vi "Binary Clock 2012 NIVerified - Cópia.vi"() -> ()   [LabVIEW 2018]
doc: "This VI displays an ultimate digital watch, which is also known as binary clock."
panel:
  out "Boolean 4":bool
  out "Boolean 3":bool
  out "Boolean 2":bool
  out "Boolean":bool
  out "'a'33 3":bool
  out "'b'33 3":bool
  out "'c'33 3":bool
  out "'d'33 3":bool
  out "'e'33 3":bool
  out "'g'33 3":bool
  out "'f'33 3":bool
  out "'a'33 2":bool
  out "'b'33 2":bool
  out "'c'33 2":bool
  out "'d'33 2":bool
  out "'e'33 2":bool
  out "'g'33 2":bool
  out "'f'33 2":bool
  out "'a'33":bool
  out "'b'33":bool
  out "'c'33":bool
  out "'d'33":bool
  out "'e'33":bool
  out "'g'33":bool
  out "'f'33":bool
  out "'a'33":bool
  out "'b'33":bool
  out "'c'33":bool
  out "'d'33":bool
  out "'e'33":bool
  out "'g'33":bool
  out "'f'33":bool
  out "'a'3 2":bool
  out "'b'3 2":bool
  out "'c'3 2":bool
  out "'d'3 2":bool
  out "'e'3 2":bool
  out "'g'3 2":bool
  out "'f'3 2":bool
  out "'e'3":bool
  out "'f'3":bool
  out "'c'3":bool
  out "'b'3":bool
  out "'d'3":bool
  out "'g'3":bool
  out "'a'3":bool
  in  "stop":bool
  in  "Lap":bool
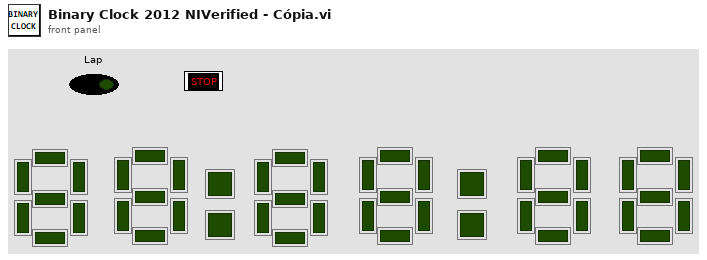
[diagram p1: front panel]
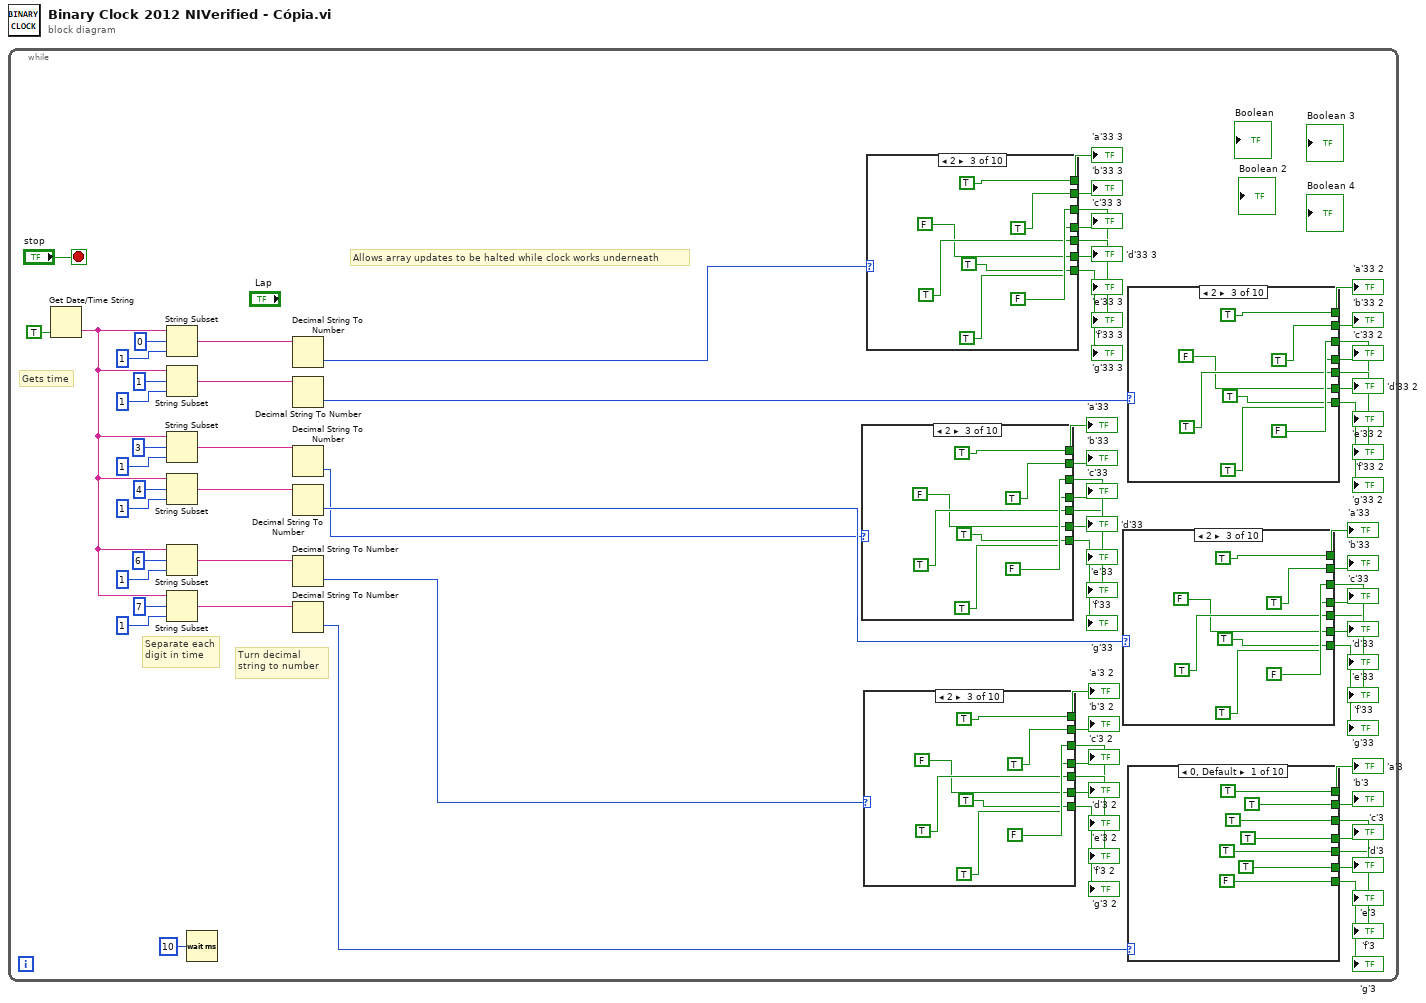
[diagram p0: block diagram]
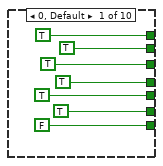
[diagram p2: hidden frame]
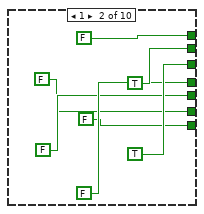
[diagram p3: hidden frame]
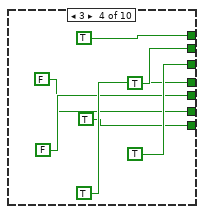
[diagram p4: hidden frame]
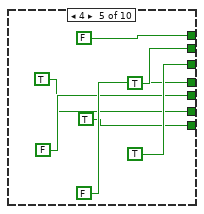
[diagram p5: hidden frame]
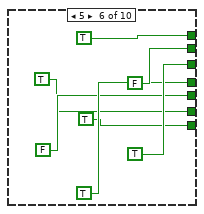
[diagram p6: hidden frame]
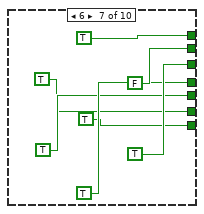
[diagram p7: hidden frame]
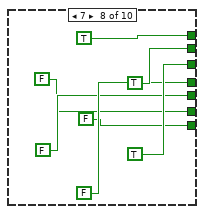
[diagram p8: hidden frame]
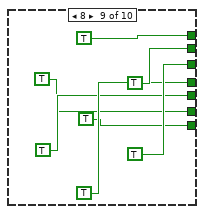
[diagram p9: hidden frame]
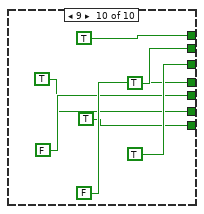
[diagram p10: hidden frame]
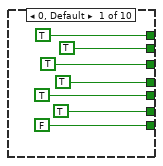
[diagram p11: hidden frame]
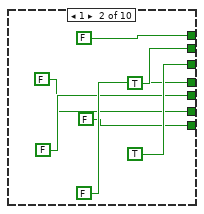
[diagram p12: hidden frame]
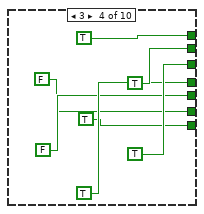
[diagram p13: hidden frame]
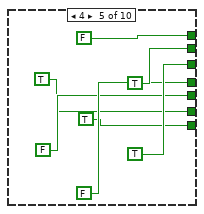
[diagram p14: hidden frame]
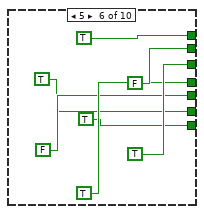
[diagram p15: hidden frame]
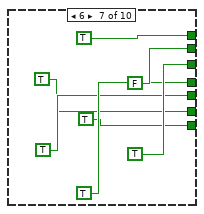
[diagram p16: hidden frame]
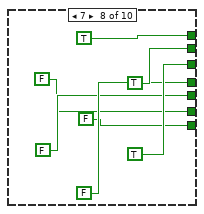
[diagram p17: hidden frame]
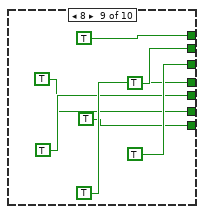
[diagram p18: hidden frame]
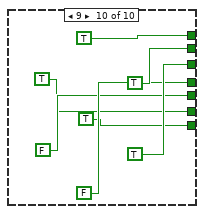
[diagram p19: hidden frame]
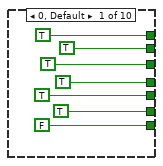
[diagram p20: hidden frame]
diagram:
  n1 = while {
    stop <- "stop" stop-if-true
    # "Allows array updates to be halted while clock works underneath"
    # "Turn decimal \nstring to number"
    # "Separate each\ndigit in time"
    # "Gets time"
    n2 = Get Date/Time String(want seconds? (F)=TRUE) -> (time string=w57:string)  [unwired: 2 in, 1 out]
    n3 = String Subset(string=w57, offset (0)=0, length (rest)=1 ("length (rest)")) -> (substring=w56:string)
    n4 = String Subset(string=w57, offset (0)=1, length (rest)=1 ("length (rest)")) -> (substring=w55:string)
    n5 = String Subset(string=w57, offset (0)=3, length (rest)=1 ("length (rest)")) -> (substring=w54:string)
    n6 = String Subset(string=w57, offset (0)=4, length (rest)=1 ("length (rest)")) -> (substring=w53:string)
    n7 = String Subset(string=w57, offset (0)=6, length (rest)=1 ("length (rest)")) -> (substring=w52:string)
    n8 = String Subset(string=w57, offset (0)=7, length (rest)=1 ("length (rest)")) -> (substring=w51:string)
    n9 = Wait (ms)(milliseconds to wait=u32 10) -> ()  [unwired: 1 out]
    n10 = Decimal String To Number(string=w56) -> (number=w1:i32)  [unwired: 2 in, 1 out]
    n11 = Decimal String To Number(string=w55) -> (number=w2:i32)  [unwired: 2 in, 1 out]
    n12 = Decimal String To Number(string=w54) -> (number=w3:i32)  [unwired: 2 in, 1 out]
    n13 = Decimal String To Number(string=w53) -> (number=w4:i32)  [unwired: 2 in, 1 out]
    n14 = Decimal String To Number(string=w52) -> (number=w33:i32)  [unwired: 2 in, 1 out]
    n15 = Decimal String To Number(string=w51) -> (number=w41:i32)  [unwired: 2 in, 1 out]
    n16 = case shown="2" w3 {
      tunnel: [TRUE ("'a'3") FALSE ("'a'3") TRUE ("'a'3") TRUE ("'a'3") FALSE ("'a'3") TRUE ("'a'3") TRUE ("'a'3") TRUE ("'a'3") TRUE ("'a'3") TRUE ("'a'3")] -> w25
      tunnel: [TRUE ("'a'3") TRUE ("'a'3") TRUE ("'a'3") TRUE ("'a'3") TRUE ("'a'3") FALSE ("'a'3") FALSE ("'a'3") TRUE ("'a'3") TRUE ("'a'3") TRUE ("'a'3")] -> w24
      tunnel: [TRUE ("'a'3") TRUE ("'a'3") FALSE ("'a'3") TRUE ("'a'3") TRUE ("'a'3") TRUE ("'a'3") TRUE ("'a'3") TRUE ("'a'3") TRUE ("'a'3") TRUE ("'a'3")] -> w23
      tunnel: [TRUE ("'a'3") FALSE ("'a'3") TRUE ("'a'3") TRUE ("'a'3") FALSE ("'a'3") TRUE ("'a'3") TRUE ("'a'3") FALSE ("'a'3") TRUE ("'a'3") FALSE ("'a'3")] -> w22
      tunnel: [TRUE ("'a'3") FALSE ("'a'3") TRUE ("'a'3") FALSE ("'a'3") FALSE ("'a'3") FALSE ("'a'3") TRUE ("'a'3") FALSE ("'a'3") TRUE ("'a'3") FALSE ("'a'3")] -> w21
      tunnel: [FALSE ("'a'3") FALSE ("'a'3") TRUE ("'a'3") TRUE ("'a'3") TRUE ("'a'3") TRUE ("'a'3") TRUE ("'a'3") FALSE ("'a'3") TRUE ("'a'3") TRUE ("'a'3")] -> w20
      tunnel: [TRUE ("'a'3") FALSE ("'a'3") FALSE ("'a'3") FALSE ("'a'3") TRUE ("'a'3") TRUE ("'a'3") TRUE ("'a'3") FALSE ("'a'3") TRUE ("'a'3") TRUE ("'a'3")] -> w19
      frame 0, Default {
      }
      frame 1 {
      }
      frame 2 {
      }
      frame 3 {
      }
      frame 4 {
      }
      frame 5 {
      }
      frame 6 {
      }
      frame 7 {
      }
      frame 8 {
      }
      frame 9 {
      }
    }
    "'a'33" <- w25
    "'b'33" <- w24
    "'c'33" <- w23
    "'d'33" <- w22
    "'e'33" <- w21
    "'g'33" <- w20
    "'f'33" <- w19
    n17 = case shown="2" w33 {
      tunnel: [TRUE ("'a'3") FALSE ("'a'3") TRUE ("'a'3") TRUE ("'a'3") FALSE ("'a'3") TRUE ("'a'3") TRUE ("'a'3") TRUE ("'a'3") TRUE ("'a'3") TRUE ("'a'3")] -> w34
      tunnel: [TRUE ("'a'3") TRUE ("'a'3") TRUE ("'a'3") TRUE ("'a'3") TRUE ("'a'3") FALSE ("'a'3") FALSE ("'a'3") TRUE ("'a'3") TRUE ("'a'3") TRUE ("'a'3")] -> w35
      tunnel: [TRUE ("'a'3") TRUE ("'a'3") FALSE ("'a'3") TRUE ("'a'3") TRUE ("'a'3") TRUE ("'a'3") TRUE ("'a'3") TRUE ("'a'3") TRUE ("'a'3") TRUE ("'a'3")] -> w36
      tunnel: [TRUE ("'a'3") FALSE ("'a'3") TRUE ("'a'3") TRUE ("'a'3") FALSE ("'a'3") TRUE ("'a'3") TRUE ("'a'3") FALSE ("'a'3") TRUE ("'a'3") FALSE ("'a'3")] -> w37
      tunnel: [TRUE ("'a'3") FALSE ("'a'3") TRUE ("'a'3") FALSE ("'a'3") FALSE ("'a'3") FALSE ("'a'3") TRUE ("'a'3") FALSE ("'a'3") TRUE ("'a'3") FALSE ("'a'3")] -> w38
      tunnel: [FALSE ("'a'3") FALSE ("'a'3") TRUE ("'a'3") TRUE ("'a'3") TRUE ("'a'3") TRUE ("'a'3") TRUE ("'a'3") FALSE ("'a'3") TRUE ("'a'3") TRUE ("'a'3")] -> w39
      tunnel: [TRUE ("'a'3") FALSE ("'a'3") FALSE ("'a'3") FALSE ("'a'3") TRUE ("'a'3") TRUE ("'a'3") TRUE ("'a'3") FALSE ("'a'3") TRUE ("'a'3") TRUE ("'a'3")] -> w40
      frame 0, Default {
      }
      frame 1 {
      }
      frame 2 {
      }
      frame 3 {
      }
      frame 4 {
      }
      frame 5 {
      }
      frame 6 {
      }
      frame 7 {
      }
      frame 8 {
      }
      frame 9 {
      }
    }
    "'a'3 2" <- w34
    "'b'3 2" <- w35
    "'c'3 2" <- w36
    "'d'3 2" <- w37
    "'e'3 2" <- w38
    "'g'3 2" <- w39
    "'f'3 2" <- w40
    n18 = case shown="2" w1 {
      tunnel: [TRUE ("'a'3") FALSE ("'a'3") TRUE ("'a'3") TRUE ("'a'3") FALSE ("'a'3") TRUE ("'a'3") TRUE ("'a'3") TRUE ("'a'3") TRUE ("'a'3") TRUE ("'a'3")] -> w5
      tunnel: [TRUE ("'a'3") TRUE ("'a'3") TRUE ("'a'3") TRUE ("'a'3") TRUE ("'a'3") FALSE ("'a'3") FALSE ("'a'3") TRUE ("'a'3") TRUE ("'a'3") TRUE ("'a'3")] -> w6
      tunnel: [TRUE ("'a'3") TRUE ("'a'3") FALSE ("'a'3") TRUE ("'a'3") TRUE ("'a'3") TRUE ("'a'3") TRUE ("'a'3") TRUE ("'a'3") TRUE ("'a'3") TRUE ("'a'3")] -> w7
      tunnel: [TRUE ("'a'3") FALSE ("'a'3") TRUE ("'a'3") TRUE ("'a'3") FALSE ("'a'3") TRUE ("'a'3") TRUE ("'a'3") FALSE ("'a'3") TRUE ("'a'3") FALSE ("'a'3")] -> w8
      tunnel: [TRUE ("'a'3") FALSE ("'a'3") TRUE ("'a'3") FALSE ("'a'3") FALSE ("'a'3") FALSE ("'a'3") TRUE ("'a'3") FALSE ("'a'3") TRUE ("'a'3") FALSE ("'a'3")] -> w9
      tunnel: [FALSE ("'a'3") FALSE ("'a'3") TRUE ("'a'3") TRUE ("'a'3") TRUE ("'a'3") TRUE ("'a'3") TRUE ("'a'3") FALSE ("'a'3") TRUE ("'a'3") TRUE ("'a'3")] -> w10
      tunnel: [TRUE ("'a'3") FALSE ("'a'3") FALSE ("'a'3") FALSE ("'a'3") TRUE ("'a'3") TRUE ("'a'3") TRUE ("'a'3") FALSE ("'a'3") TRUE ("'a'3") TRUE ("'a'3")] -> w11
      frame 0, Default {
      }
      frame 1 {
      }
      frame 2 {
      }
      frame 3 {
      }
      frame 4 {
      }
      frame 5 {
      }
      frame 6 {
      }
      frame 7 {
      }
      frame 8 {
      }
      frame 9 {
      }
    }
    "'a'33 3" <- w5
    "'b'33 3" <- w6
    "'c'33 3" <- w7
    "'d'33 3" <- w8
    "'e'33 3" <- w9
    "'g'33 3" <- w10
    "'f'33 3" <- w11
    n19 = case shown="2" w4 {
      tunnel: [TRUE ("'a'3") FALSE ("'a'3") TRUE ("'a'3") TRUE ("'a'3") FALSE ("'a'3") TRUE ("'a'3") TRUE ("'a'3") TRUE ("'a'3") TRUE ("'a'3") TRUE ("'a'3")] -> w32
      tunnel: [TRUE ("'a'3") TRUE ("'a'3") TRUE ("'a'3") TRUE ("'a'3") TRUE ("'a'3") FALSE ("'a'3") FALSE ("'a'3") TRUE ("'a'3") TRUE ("'a'3") TRUE ("'a'3")] -> w31
      tunnel: [TRUE ("'a'3") TRUE ("'a'3") FALSE ("'a'3") TRUE ("'a'3") TRUE ("'a'3") TRUE ("'a'3") TRUE ("'a'3") TRUE ("'a'3") TRUE ("'a'3") TRUE ("'a'3")] -> w30
      tunnel: [TRUE ("'a'3") FALSE ("'a'3") TRUE ("'a'3") TRUE ("'a'3") FALSE ("'a'3") TRUE ("'a'3") TRUE ("'a'3") FALSE ("'a'3") TRUE ("'a'3") FALSE ("'a'3")] -> w29
      tunnel: [TRUE ("'a'3") FALSE ("'a'3") TRUE ("'a'3") FALSE ("'a'3") FALSE ("'a'3") FALSE ("'a'3") TRUE ("'a'3") FALSE ("'a'3") TRUE ("'a'3") FALSE ("'a'3")] -> w28
      tunnel: [FALSE ("'a'3") FALSE ("'a'3") TRUE ("'a'3") TRUE ("'a'3") TRUE ("'a'3") TRUE ("'a'3") TRUE ("'a'3") FALSE ("'a'3") TRUE ("'a'3") TRUE ("'a'3")] -> w27
      tunnel: [TRUE ("'a'3") FALSE ("'a'3") FALSE ("'a'3") FALSE ("'a'3") TRUE ("'a'3") TRUE ("'a'3") TRUE ("'a'3") FALSE ("'a'3") TRUE ("'a'3") TRUE ("'a'3")] -> w26
      frame 0, Default {
      }
      frame 1 {
      }
      frame 2 {
      }
      frame 3 {
      }
      frame 4 {
      }
      frame 5 {
      }
      frame 6 {
      }
      frame 7 {
      }
      frame 8 {
      }
      frame 9 {
      }
    }
    "'a'33" <- w32
    "'b'33" <- w31
    "'c'33" <- w30
    "'d'33" <- w29
    "'e'33" <- w28
    "'g'33" <- w27
    "'f'33" <- w26
    n20 = case shown="2" w2 {
      tunnel: [TRUE ("'a'3") FALSE ("'a'3") TRUE ("'a'3") TRUE ("'a'3") FALSE ("'a'3") TRUE ("'a'3") TRUE ("'a'3") TRUE ("'a'3") TRUE ("'a'3") TRUE ("'a'3")] -> w12
      tunnel: [TRUE ("'a'3") TRUE ("'a'3") TRUE ("'a'3") TRUE ("'a'3") TRUE ("'a'3") FALSE ("'a'3") FALSE ("'a'3") TRUE ("'a'3") TRUE ("'a'3") TRUE ("'a'3")] -> w13
      tunnel: [TRUE ("'a'3") TRUE ("'a'3") FALSE ("'a'3") TRUE ("'a'3") TRUE ("'a'3") TRUE ("'a'3") TRUE ("'a'3") TRUE ("'a'3") TRUE ("'a'3") TRUE ("'a'3")] -> w14
      tunnel: [TRUE ("'a'3") FALSE ("'a'3") TRUE ("'a'3") TRUE ("'a'3") FALSE ("'a'3") TRUE ("'a'3") TRUE ("'a'3") FALSE ("'a'3") TRUE ("'a'3") FALSE ("'a'3")] -> w15
      tunnel: [TRUE ("'a'3") FALSE ("'a'3") TRUE ("'a'3") FALSE ("'a'3") FALSE ("'a'3") FALSE ("'a'3") TRUE ("'a'3") FALSE ("'a'3") TRUE ("'a'3") FALSE ("'a'3")] -> w16
      tunnel: [FALSE ("'a'3") FALSE ("'a'3") TRUE ("'a'3") TRUE ("'a'3") TRUE ("'a'3") TRUE ("'a'3") TRUE ("'a'3") FALSE ("'a'3") TRUE ("'a'3") TRUE ("'a'3")] -> w17
      tunnel: [TRUE ("'a'3") FALSE ("'a'3") FALSE ("'a'3") FALSE ("'a'3") TRUE ("'a'3") TRUE ("'a'3") TRUE ("'a'3") FALSE ("'a'3") TRUE ("'a'3") TRUE ("'a'3")] -> w18
      frame 0, Default {
      }
      frame 1 {
      }
      frame 2 {
      }
      frame 3 {
      }
      frame 4 {
      }
      frame 5 {
      }
      frame 6 {
      }
      frame 7 {
      }
      frame 8 {
      }
      frame 9 {
      }
    }
    "'a'33 2" <- w12
    "'b'33 2" <- w13
    "'c'33 2" <- w14
    "'d'33 2" <- w15
    "'e'33 2" <- w16
    "'g'33 2" <- w17
    "'f'33 2" <- w18
    n21 = case shown="0, Default" w41 {
      tunnel: [TRUE ("'a'3") FALSE ("'a'3") TRUE ("'a'3") TRUE ("'a'3") FALSE ("'a'3") TRUE ("'a'3") TRUE ("'a'3") TRUE ("'a'3") TRUE ("'a'3") TRUE ("'a'3")] -> w48
      tunnel: [TRUE ("'a'3") TRUE ("'a'3") TRUE ("'a'3") TRUE ("'a'3") TRUE ("'a'3") FALSE ("'a'3") FALSE ("'a'3") TRUE ("'a'3") TRUE ("'a'3") TRUE ("'a'3")] -> w47
      tunnel: [TRUE ("'a'3") TRUE ("'a'3") FALSE ("'a'3") TRUE ("'a'3") TRUE ("'a'3") TRUE ("'a'3") TRUE ("'a'3") TRUE ("'a'3") TRUE ("'a'3") TRUE ("'a'3")] -> w46
      tunnel: [TRUE ("'a'3") FALSE ("'a'3") TRUE ("'a'3") TRUE ("'a'3") FALSE ("'a'3") TRUE ("'a'3") TRUE ("'a'3") FALSE ("'a'3") TRUE ("'a'3") FALSE ("'a'3")] -> w45
      tunnel: [TRUE ("'a'3") FALSE ("'a'3") TRUE ("'a'3") FALSE ("'a'3") FALSE ("'a'3") FALSE ("'a'3") TRUE ("'a'3") FALSE ("'a'3") TRUE ("'a'3") FALSE ("'a'3")] -> w44
      tunnel: [FALSE ("'a'3") FALSE ("'a'3") TRUE ("'a'3") TRUE ("'a'3") TRUE ("'a'3") TRUE ("'a'3") TRUE ("'a'3") FALSE ("'a'3") TRUE ("'a'3") TRUE ("'a'3")] -> w43
      tunnel: [TRUE ("'a'3") FALSE ("'a'3") FALSE ("'a'3") FALSE ("'a'3") TRUE ("'a'3") TRUE ("'a'3") TRUE ("'a'3") FALSE ("'a'3") TRUE ("'a'3") TRUE ("'a'3")] -> w42
      frame 0, Default {
      }
      frame 1 {
      }
      frame 2 {
      }
      frame 3 {
      }
      frame 4 {
      }
      frame 5 {
      }
      frame 6 {
      }
      frame 7 {
      }
      frame 8 {
      }
      frame 9 {
      }
    }
    "'a'3" <- w48
    "'b'3" <- w47
    "'c'3" <- w46
    "'d'3" <- w45
    "'e'3" <- w44
    "'g'3" <- w43
    "'f'3" <- w42
  }
